vi "3-2.vi"() -> ()   [LabVIEW 2014]
panel:
  out "# of Iterations":dbl
  out "Current Number":dbl
  in  "Numeric":dbl
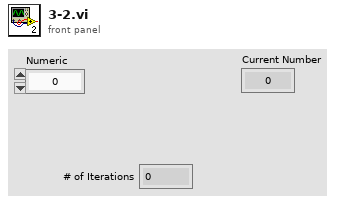
[diagram p1: front panel]
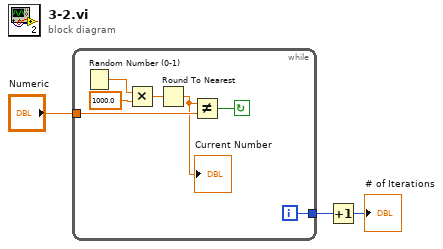
[diagram p0: block diagram]
diagram:
  n1 = while {
    tunnel: [w10] -> w3
    tunnel: "Numeric" -> [w9]
    i -> [w10]
    stop <- w4 continue-if-true
    n2 = Random Number (0-1)() -> (number: 0 to 1=w8:dbl)
    n3 = Multiply(x=w8, y=1000.0) -> (x*y=w6:dbl)
    n4 = Round To Nearest(number=w6) -> (nearest integer value=w5:dbl)
    "Current Number" <- w5
    n5 = Not Equal?(x=w5, y=w9) -> (x != y?=w4:bool)
  }
  n6 = Increment(x=w3) -> (x+1=→"# of Iterations":i32)
